vi "Insert Into Array (String).vi"(9 "index":i32, 10 "String":string, 11 "JSON Value in":refnum<class "JSON Value.lvclass">) -> (3 "JSON Value out":refnum<class "JSON Value.lvclass">)   [LabVIEW 2016, in "JSON Value.lvclass"]
doc: "Inserts an element or subarray into a JSON array at the point you specify in index."
uses:
  JSON Value.lvclass
  Insert Into Array (Value).vi
  New JSON Value/New JSON (String).vi
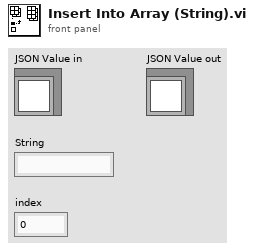
[diagram p1: front panel]
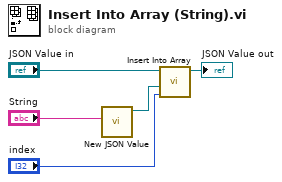
[diagram p0: block diagram]
diagram:
  n1 = call-poly "New JSON Value.vi"("value"="String") -> ("JSON Value out"=w2:refnum<class "JSON Value.lvclass">)  [unwired: 9 in, 1 out]
  n2 = call-poly "Insert Into Array.vi"("index"="index", 9:"JSON Value in"=w2, 11:"JSON Value in"="JSON Value in") -> ("JSON Value out"=→"JSON Value out":refnum<class "JSON Value.lvclass">)  [unwired: 8 in]
